vi "PID 1D Correction.vi"(1 "In Range?":bool, 2 "Distance off":dbl, 3 "PID Booleans":cluster{"PID Off?":bool, "Invert value":bool}, 4 "PID inputs":T1={"output range"={"high"=100.0, "low"=-100.0}, "PID gains"={"proportional gain (Kp)"=1.0, "integral time (Ki)"=0.0, "derivative time (Kd)"=0.0}} {"output range"."low" format="%.2f"; "output range"."high" format="%.2f"; "PID gains"."derivative time (Kd)" format="%.3f"; "PID gains"."integral time (Ki)" format="%.3f"; "PID gains"."proportional gain (Kp)" format="%.3f"}) -> (0 "Correction":dbl)   [LabVIEW 2023]
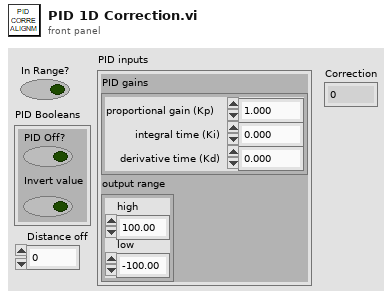
[diagram p1: front panel]
types:
  T1 = cluster{"output range":cluster{"high":dbl, "low":dbl}, "PID gains":cluster{"proportional gain (Kp)":dbl, "integral time (Ki)":dbl, "derivative time (Kd)":dbl}}
  T2 = cluster{"proportional gain (Kp)":dbl, "integral time (Ki)":dbl, "derivative time (Kd)":dbl}
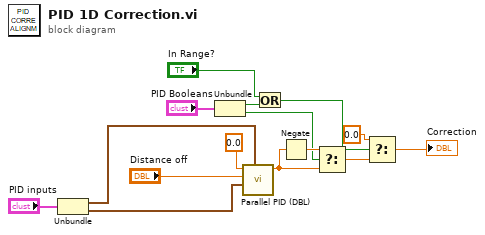
[diagram p0: block diagram]
diagram:
  n1 = Unbundle("PID inputs") -> ("output range"=w11:cluster{"high":dbl, "low":dbl}, "PID gains"=w10:T2)
  n2 = Unbundle("PID Booleans") -> ("PID Off?"=w3:bool, "Invert value"=w7:bool)
  n3 = call <vilib>:"Parallel PID (DBL).vi"("output range"=w11, "PID gains"=w10, "process variable"="Distance off", "setpoint"=0.0) -> ("output"=w13:dbl)  [unwired: 4 in, 3 out]
  n4 = Or(x="In Range?", y=w3) -> (x .or. y?=w2:bool)
  n5 = Negate(x=w13) -> (-x=w14:dbl)
  n6 = Select(t=w14, s=w7, f=w13) -> (s? t:f=w9:dbl)
  n7 = Select(t=0.0, s=w2, f=w9) -> (s? t:f=→"Correction":dbl)
